vi "Run next.vi"(10 "Boolean 2":bool, 11 "Boolean":bool) -> (3 "Enum":T1)   [LabVIEW 2014]
doc: "Calcul next step"
uses:
  Enum.ctl
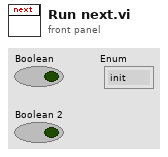
[diagram p1: front panel]
types:
  T1 = typedef "Enum.ctl" = enum16{"init", "run", "close"}
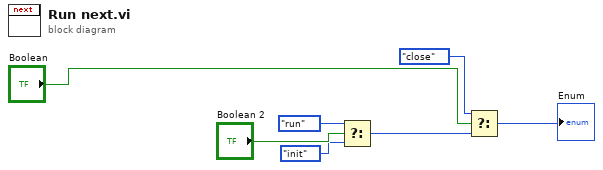
[diagram p0: block diagram]
diagram:
  n1 = Select(t=Enum."run", s="Boolean 2", f=Enum."init") -> (s? t:f=w5:T1)
  n2 = Select(t=Enum."close", s="Boolean", f=w5) -> (s? t:f=→"Enum":T1)
